vi "ParseIVFolder.vi"(8 "error in (no error)":errorcluster, 11 "File or Folder Path":path=path "B:/SketchSET/SA03008H.20180718/21-BG+SG_Sweep+OVERNIGHT") -> (0 "error out":errorcluster, 3 "output cluster":T1)   [LabVIEW 2016]
uses:
  <vilib>/Analysis/NI_AALPro.lvlib
  <vilib>/Analysis/polynomials.llb/Unique Numbers and Multiplicity (DBL).vi
panel:
  in  "# of fields/Temperatures":i32=1
  in  "Field Period":i32=1
  in  "Additional comments":string
  in  "IV setup":T2={"# of Vslow"=101, "# Vfast"=41, "#IV Curves at each gate"=1, "B/T offset"=0, "Discard first # curves"=0, "Manual offset"=0}
  in  "Scan names":string[](array[string])=["DSA_Vsg1", "B", "B"]
  in  "Portion of data":cluster{dbl, dbl}(slide)={1.0, 0.0} scale=0.0..1.0
  in  "Decimate point":dbl=10.0 format="%#_1f"
  in  "T/B     third axis":bool
  in  "Extract parameters from comments?":bool=TRUE
  in  "index 2":T3={"A"=3, "B"=5, "C"=3, "D"=5, "E"=3, "N1"=2, "N2"=2, "N3"=3, "N4"=4, "A 1"=3, "A 2"=3, "C 1"=3, "C 2"=3, "E 2"=4}
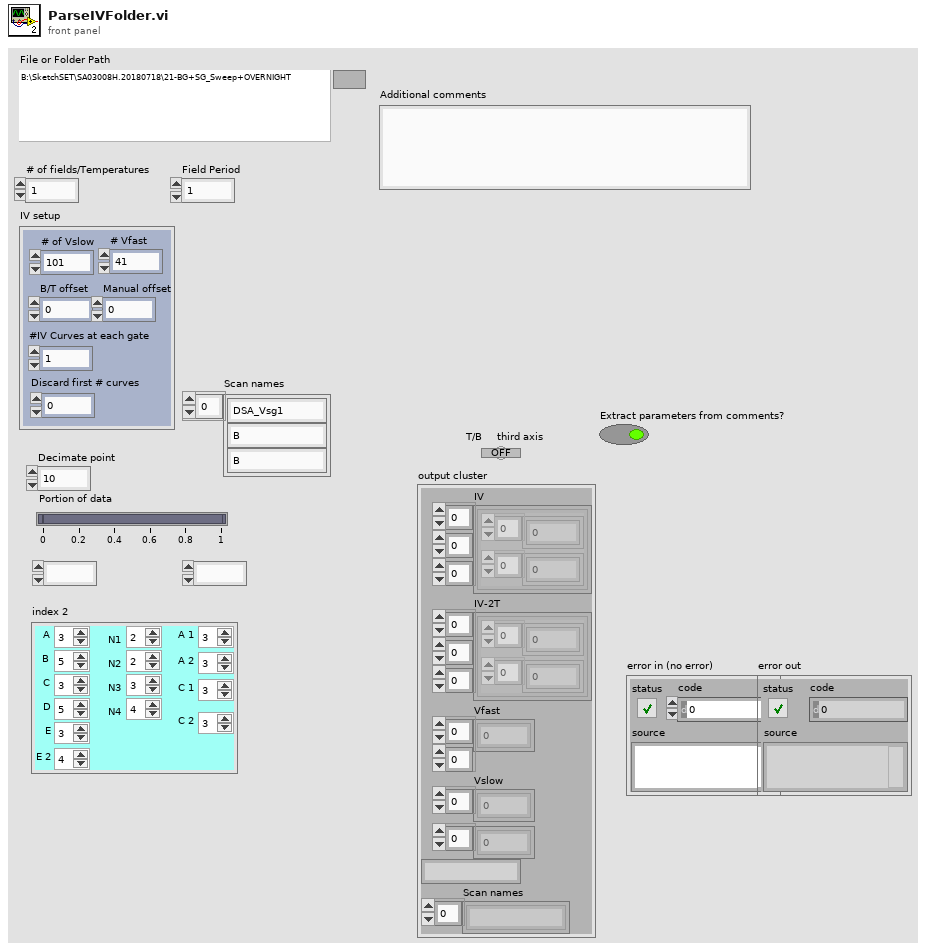
[diagram p1: front panel]
types:
  T1 = cluster{"IV":cluster{dbl[], dbl[]}[][][], "IV-2T":cluster{dbl[], dbl[]}[][][], "Vfast":dbl[][], "Vslow":dbl[], dbl[], string, "Scan names":string[]}
  T2 = cluster{"# of Vslow":i32, "# Vfast":i32, "#IV Curves at each gate":i32, "B/T offset":i32, "Discard first # curves":i32, "Manual offset":i32}
  T3 = cluster{"A":i32, "B":i32, "C":i32, "D":i32, "E":i32, "N1":i32, "N2":i32, "N3":i32, "N4":i32, "A 1":i32, "A 2":i32, "C 1":i32, "C 2":i32, "E 2":i32}
  T4 = typedef "SweepControl.lvclass/ScanControl.ctl" = T5[]
  T5 = typedef "SweepControl.lvclass/Cluster - ScanControl.ctl" = cluster{"Priority":T6, "Scan name":T7}
  T6 = typedef "SweepControl.lvclass/Enum - Priority.ctl" = enum16{"Priority 0", "Priority 1", "Priority 2", "Priority 3", "Priority 4", "Priority 5"}
  T7 = typedef "SweepControl.lvclass/Enum - Action.ctl" = enum16{"OFF", "DSA_Vamp", "DSA_freq", "DSA_Vsg1", "DSA_Vsg2", "DSA_Vsg3", "DAQ_Vbg", "B_Field", "Humidity", "Temp", "MW_freq1", "MW_freq2", "MW_amplitude1", "MW_amplitude2"}
  T8 = typedef "SweepControl.lvclass/ScanParamters.ctl" = T9[]
  T9 = typedef "SweepControl.lvclass/Cluster - ScanParamters.ctl" = cluster{"Start":dbl, "End":dbl, "Step":dbl, "Rate":dbl, "wait (ms)":u32, "address":refnum<visa-resource-name>, "Channel":i32}
  T10 = cluster{"Sorted scan control":cluster{T4}[], "Sorted scan parameters":cluster{T8}[], "# Of Sweep Pts. Fast to Slow":i16[]}
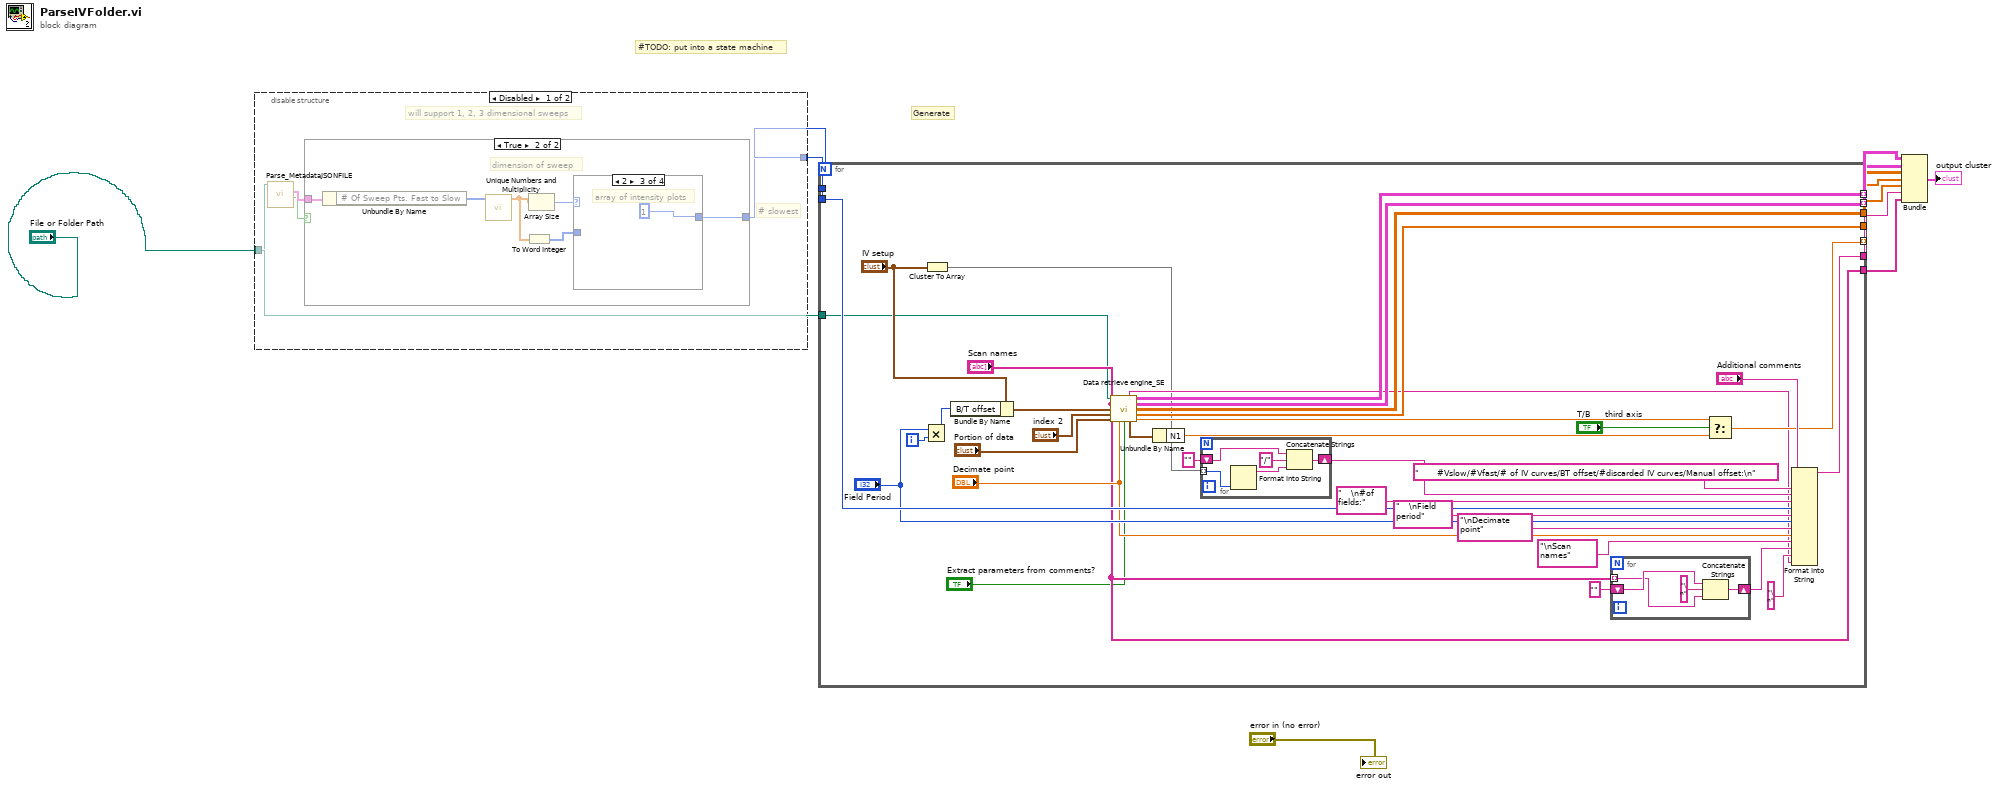
[diagram p0: block diagram]
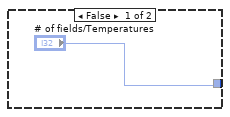
[diagram p2: hidden frame]
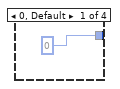
[diagram p3: hidden frame]
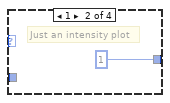
[diagram p4: hidden frame]
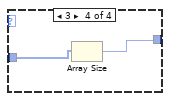
[diagram p5: hidden frame]
diagram:
  # "#TODO: put into a state machine"
  # "Generate"
  n1 = disable-structure shown="Disabled" {
    disable-tunnel: [w14 _] -> w4
    disable-tunnel: "File or Folder Path" -> [w12 _]
    frame Disabled {
      # "will support 1, 2, 3 dimensional sweeps"
      # "# slowest"
      n2 = call "Parse_MetadataJSONFILE.vi"("File or Folder Path"=w12) -> ("file or folder exists?"=w13:bool, "output cluster"=w15:T10)  [unwired: 8 in, 1 out]
      n3 = case shown="True" w13 {
        tunnel: w15 -> [_ w22]
        tunnel: ["# of fields/Temperatures" w19] -> w14
        frame False {
        }
        frame True {
          # "dimension of sweep"
          n4 = Unbundle By Name(w22) -> ("# Of Sweep Pts. Fast to Slow"=w21:i16[])
          n5 = call-poly <vilib>:"Unique Numbers and Multiplicity.vi"("Numbers"=w21) -> ("Unique Numbers"=w18:dbl[])  [unwired: 8 in, 2 out]
          n6 = To Word Integer(number=w18) -> (16bit integer=w17:i16[])
          n7 = Array Size(array=w18) -> (size(s)=w20:i32)
          n8 = case shown="2" w20 {
            tunnel: [0 1 1 w27] -> w19
            tunnel: w17 -> [_ _ _ w26]
            frame 0, Default {
            }
            frame 1 {
              # "Just an intensity plot"
            }
            frame 2 {
              # "array of intensity plots"
            }
            frame 3 {
              n9 = Array Size(array=w26) -> (size(s)=w27:i32)
            }
          }
        }
      }
    }
    frame Enabled {
    }
  }
  n10 = for {
    N: w4 -> [_]
    tunnel: [w62] -> w11 mode=indexing
    tunnel: [w58] -> w8
    tunnel: [w57] -> w7
    tunnel: [w56] -> w10 mode=indexing
    tunnel: [w39] -> w6 mode=indexing
    tunnel: w4 -> [_]
    tunnel: w4 -> [w47]
    tunnel: [w38] -> w9
    tunnel: ["Scan names"] -> w5
    tunnel: "File or Folder Path" -> [w29]
    i -> [w61]
    n11 = Multiply(x="Field Period", y=w61) -> (x*y=w59:i32)
    n12 = Cluster To Array(cluster="IV setup") -> (array=w28:i32[])
    n13 = Bundle By Name(cluster="IV setup", "B/T offset"=w59) -> (w52:T2)
    n14 = call "Data retrieve engine_SE.vi"("File or Folder Path"=w29, "Scan names"="Scan names", "IV setup"=w52, "index"="index 2", "Portion of data"="Portion of data", "Decimate point"="Decimate point", "Extract paramaters from comments?"="Extract parameters from comments?") -> ("Comments"=w33:string, "IV"=w62:cluster{dbl[], dbl[]}[][], "IV-2T"=w56:cluster{dbl[], dbl[]}[][], "Vfast"=w58:dbl[][], "Vslow"=w57:dbl[], "N"=w60:cluster{"N1":dbl, "N2":dbl, "N3":dbl, "N4":dbl}, "Vslowest"=w42:dbl)  [unwired: 2 in]
    n15 = Unbundle By Name(w60) -> ("N1"=w41:dbl)
    n16 = for {
      tunnel: w28 -> [w71] mode=indexing
      shift-right: [w68] -> w49
      shift-left: "" -> [w67]
      n17 = Format Into String(w71) -> (resulting string=w70:string)  [unwired: 3 in, 1 out]
      n18 = Concatenate Strings(w67, "/" ("string"), w70) -> (w68:string)
    }
    n19 = for {
      tunnel: "Scan names" -> [w64] mode=indexing
      shift-right: [w66] -> w35
      shift-left: "" -> [w65]
      n20 = Concatenate Strings(w65, "\n" ("string"), w64) -> (w66:string)
    }
    n21 = Select(t=w42, s="T/B     third axis", f=w41) -> (s? t:f=w39:dbl)
    n22 = Format Into String(initial string="Additional comments", "      #Vslow/#Vfast/# of IV curves/BT offset/#discarded IV curves/Manual offset:\n" ("string"), w49, "   \n#of fields:" ("string"), w47, "   \nField period" ("string"), "Field Period", "\nDecimate point", "Decimate point", "\nScan names", w35, "\n" ("input 11"), w33) -> (resulting string=w38:string)  [unwired: 2 in, 1 out]
  }
  n23 = Bundle("IV"=w11, "IV-2T"=w10, "Vfast"=w8, "Vslow"=w7, w6, w9, "Scan names"=w5) -> (→"output cluster":T1)  [unwired: 1 in]
  "error out" <- "error in (no error)"
